vi "ResFileRigExcluder.vi"(7 "Rig Name":string="WT1", 10 "Rig Exclusion Filepath":path=path "/Volumes/CentralDataCache/Projects/GO69T1/Results/KAG69/RigExclusion.xls", 11 "Results file":path=path "/Volumes/CentralDataCache/Projects/GO69T1/Results/KAG69/Profiles2016-08 copy.xls") -> (3 "New Filepath":path=path "/Volumes/CentralDataCache/Projects/GO69T1/Results/KAG69/Profiles2016-08 copy_RigSpec.xls")   [LabVIEW 2016]
doc: "Given {complete Res File, Rig Name, Rig Exclusion Filepath}, this VI returns a Rig-Specific Results File.\n< Rig Name > = relevant Rig Name ; \n< Results File > = comprehensive Results File ; \n< Rig Exclusion Filepath > = path to text file containing list of all Rigs at facility ; \n< New Filepath > = Rig-Specific Results File contains all generic metadata, measurements, and data pertaining to < Rig Name >"
uses:
  Anemometry Sub Vis/Data_plotting_vis/Data_File_Type.ctl
  <vilib>/Utility/file.llb/Read Delimited Spreadsheet (string).vi
  <vilib>/regexp/Match Regular Expression.xnode
panel:
  out "Desired Channels":string[](array[string])=["Date:of:Measurement", "Time:Measurement:Commenced", "Seconds:since:1st Jan", "Measuring:Instrument:Type", "User:Comments:", "Run:Messages:", "Raw:Data:Filename", "Pitot (Uref):X Position:X (mm)", "Pitot (Uref):Y Position:Y (mm)", "Pitot (Uref):Z Position:Z (mm)", "Pitot (Uref):Mean:UREF", "Pitot (Uref):Variance:uref^2", "Pitot (Uref):Standard Error:in Mean", "Pitot (Uref):Timescale Estimate:Integrated to 25%", "Pitot (Uref):Calibration:Filename", "HW (Uhf):X Position:X (mm)", "HW (Uhf):Y Position:Y (mm)", "HW (Uhf):Z Position:Z (mm)", "HW (Uhf):Mean:UHF", "HW (Uhf):Variance:uhf^2", "HW (Uhf):Skewness:uhf^3/(uhf^2)^1.5", "HW (Uhf):Kurtosis:(uhf^4/(uhf^2)^2) -3", "HW (Uhf):Standard Error:in Mean", "HW (Uhf):Standard Error:in Variance", "HW (Uhf):Timescale Estimate:Integrated to 25%", "HW (Uhf):Calibration:Filename", "HW (Uhf):Calibration:Drift", "HW (Uhf):Calibration:Interval", "Av Analogue:Sampling:Rate", "No of:Analogue:Samples", "No Of:Measurement:Blocks", "Flow:Measurement:Time", "Reference:Temperature:Used for Corrections", "Atmos:Pressure:Used for Corrections", "Multi Run:Command:Filename", "Multi Run:Start Time:", "Multi Run:Duration in:Minutes", "Multi Run:Row:Type", "Multi Run:Row:Number", "Multi Run:Extra:Command", "Prog Post:Process:Mode", "Acquisition:PlugIn:Used", "Original:Results:Filename", "Time:According:to", "Client:Seconds:Since", "Averaging:Period:Used", "ADAM:Scan:Time", "Complete:Scan:Period", "Status:of:MetadataSys", "Status:of:Post_Processing_Machine", "CSU:Pressure:mBar", "CSU:Pressure:Age_min", "CFWS:Pressure:mBar", "CFWS:Pressure:Age_min", "CS:AvgPressure:mBar", "WT1:StaticP:0", "WT1:StaticP:1", "WT1:StaticP:2", "WT1:StaticP:3", "WT1:StaticP:4", "WT1:StaticP:5", "WT1:StaticP:6", "WT1:StaticP:7", "WT1:AvStat:P0", "WT1:AvStat:P1", "WT1:AvStat:P2", "WT1:AvStat:P3", "WT1:AvStat:P4", "WT1:AvStat:P5", "WT1:AvStat:P6", "WT1:AvStat:P7", "WT1:Temperature:C", "WT1:Motor:Enable", "WT1:Speed:Calib Tweak", "WT1:Speed:Dem Velocity", "WT1:Speed:Dem Voltage", "WT1:Speed:Meas Velocity", "WT1:Speed:Send Voltage", "WT1:VFD:FREQ", "WT1:RoofSetting:Pressures", "WT1:RoofSetting:Heights", "WT1:Turntable:Azimuth", "WT1Traverse:Motor:X", "WT1Traverse:Motor:Y", "WT1Traverse:Motor:Z", "WT1:Z:Corrections", "WT1 MD:User:Name", "WT1 MD:Project:Number", "WT1 MD:Project:Configuration", "WT1 MD:Pitot:Height", "WT1 MD:Pitot:X-location", "WT1 MD:Roughness:Type", "WT1 MD:Roughness:Size", "WT1 MD:Roughness:AdditionalElements", "WT1 MD:Trip:Height", "WT1 MD:Trip:Location", "WT1 MD:Spires:Type", "WT1 MD:Spires:Code", "WT1 MD:Spires:FullCount", "WT1 MD:Spires:HalfCount", "WT1 MD:Spires:Location", "WT1 MD:Spires:Height", "WT1 MD:Spires:TopWidth", "WT1 MD:Spires:BaseWidth", "WT1 MD:Comments:", "WT1:AQ MD:SourceID", "WT1:Cal Gas:Selector", "WT1:Cal Gas 1:BottleID", "WT1:Cal Gas 1:GasMixture", "WT1:Cal Gas 1:Conc", "WT1:Cal Gas 2:BottleID", "WT1:Cal Gas 2:GasMixture", "WT1:Cal Gas 2:Conc", "WT1:Cal Gas 3:BottleID", "WT1:Cal Gas 3:GasMixture", "WT1:Cal Gas 3:Conc", "WT1:Autozero:Pressures", "ADAM:Scan:Pacer", "WT1:rho:(kg/m^3)", "WT1:FID:IP", "WT1:MFC32:Read%", "WT1:MFC31:Read%", "WT1:MFC25:Read%", "WT1:MFC21:Read%", "WT1:MFC13:Read%", "WT1:MFC12:Read%", "WT1:MFC:Enable", "Status:of:WT1", "WT1 Metadata:Roughness:Notes", "ADAM:Scan:Comments", "Client:ADAM:Scan", "::", "::1904", "::", "::", "::", "::Inc Path", "::", "::", "::", "::", "::", "::Not %", "::(s)", "::", "::", "::", "::", "::", "::", "::", "::", "::Not %", "::Not %", "::(s)", "::", "::%", "::Minutes", "::Freq (Hz)", "::Per Block", "::", "::(mins)", "::", "::", "::", "::", "::", "::", "::", "::", "::", "::", "::", "::Client", "::1st Jan 1904", "::Seconds", "::CPP-ScanTimeKeeper.vi", "::sec", "::", "::", "::", "::CSUWebClient.vi", "::", "::CFWSWebClient.vi", "::", "::CSPressureSelector.vi", "::", "::", "::", "::", "::", "::", "::", "::", ":: WT1", ":: WT1", ":: WT1", ":: WT1", ":: WT1", ":: WT1", ":: WT1", ":: WT1", "::", "::LabJackT7.vi", "::", "::", "::WT1", "::WT1", "::", "::", "::", "::", "::", "::", "::", "::", "::", "::", "::", "::None", "::1000.0 mm", "::-3350.0 mm", "::0.0-mm None + None", "::0.0-mm None", "::98", "::0.0 mmModified 09-08-2016 21", "::0.0 mm", "::Irwin", "::24X4", "::0 full", "::0 half", "::0.0 mm", "::609.6 mm", "::0.0 mm", "::101.6 mm", "::NEW 1.5in roughness", "::", "::", "::", "::", "::", "::", "::", "::", "::", "::", "::", "::", "::", "::", "::", "::", "::", "::", "::", "::", "::", "::", "::", "::", "::", "::", "::", "::", "::", "::", "::", "::", "::", "::UINT16", "::UINT16", "::UINT16", "::UINT16", "::UINT16", "::UINT16", "::UINT16", "::UINT16", "::", "::", "::", "::", "::", "::", "::", "::", "::", "::", "::", "::", "::", "::", "::", "::", "::", "::", "::", "::A", "::1000.0 mm", "::-3532.0 mm", "::50.8-mm Cubes + 98", "::50.8-mm Cubes", "::98", "::558.8 mm", "::527.0 mm", "::Irwin", "::72X5", "::4 full", "::2 half", "::223.8 mm", "::1828.8 mm", "::44.4 mm", "::133.3 mm", "::(add comments)", "::", "::", "::100.00 inches", "::200.00 inches", "::100.00 inches", "::-50.00 inches", "::0.00 inches", "::RE-run of 413... this time with gases on!! (10x20x10cm EBD w/ stack in center)", "::", "::", "::", "::", "::", "::", "::", "::", "::", "::", "::", "::", "::", "::", "::", "::", "::", "::", "::", "::", "::", "::", "::", "::", "::", "::", "::A", "::1000.0 mm", "::-3532.0 mm", "::50.8-mm Cubes + 98", "::50.8-mm Cubes", "::98", "::558.8 mm", "::527.0 mm", "::Irwin", "::72X5", "::4 full", "::2 half", "::223.8 mm", "::1828.8 mm", "::44.4 mm", "::133.3 mm", "::(add comments)", "::", "::", "::", "::", "::", "::", "::", "::", "::", "::", "::", "::", "::", "::", "::", "::", "::", "::", "::", "::", "::", "::", "::", "::", "::", "::", "::", "::", "::", "::", "::", "::", "::", "::", "::", "::", "::", "::", "::", "::", "::", "::", "::Xdim", "::Ydim (mm)", "::Zdim (mm)", "::(mm)", "::(mm)", "::", "::(add comments)", "::", "::", "::", "::", "::", "::", "::", "::", "::", "::", "::", "::", "::", "::", "::", "::", "::", "::", "::", "::", "::", "::", "::", "::", "::", "::", "::", "::", "::Fr Server", "::Comments"]
  out "Desired Columns":i32[](array[numeric])=[0, 1, 2, 3, 4, 5, 6, 7, 8, 9, 10, 11, 12, 13, 14, 15, 16, 17, 18, 19, 20, 21, 22, 23, 24, 25, 26, 27, 28, 29, 30, 31, 32, 33, 34, 35, 36, 37, 38, 39, 40, 41, 42, 43, 44, 45, 46, 47, 48, 49, 51, 52, 53, 54, 55, 56, 57, 58, 59, 60, 61, 62, 63, 64, 65, 66, 67, 68, 69, 70, 71, 72, 73, 74, 75, 76, 77, 78, 79, 80, 81, 82, 83, 84, 85, 86, 87, 88, 89, 90, 91, 92, 93, 94, 95, 96, 97, 98, 99, 100, 101, 102, 103, 104, 105, 106, 107, 108, 109, 110, 111, 112, 113, 114, 115, 116, 261, 266, 285, 287, 298, 299, 300, 301, 302, 303, 304, 322, 323, 324, 325, 326, 327, 328, 329, 330, 331, 332, 333, 334, 335, 336, 337, 338, 339, 340, 341, 342, 343, 344, 345, 346, 347, 348, 349, 350, 351, 352, 353, 354, 355, 356, 357, 358, 359, 360, 361, 362, 363, 364, 365, 366, 367, 368, 369, 370, 371, 372, 373, 374, 375, 376, 377, 378, 379, 380, 381, 382, 383, 384, 385, 386, 387, 388, 389, 390, 391, 392, 393, 394, 395, 396, 397, 398, 399, 400, 401, 402, 403, 404, 405, 406, 407, 408, 409, 410, 411, 412, 413, 414, 415, 416, 417, 418, 419, 420, 421, 422, 423, 424, 425, 426, 427, 428, 429, 430, 431, 432, 433, 434, 435, 436, 437, 438, 439, 440, 441, 442, 443, 444, 445, 446, 447, 448, 449, 450, 451, 462, 463, 464, 465, 468, 469, 470, 471, 472, 473, 474, 475, 476, 477, 478, 479, 480, 481, 482, 483, 484, 485, 486, 487, 488, 489, 490, 491, 492, 493, 494, 495, 496, 497, 498, 499, 500, 501, 502, 503, 504, 505, 506, 507, 508, 509, 510, 511, 512, 513, 514, 515, 516, 517, 518, 519, 520, 521, 522, 523, 524, 525, 526, 527, 528, 529, 530, 531, 532, 533, 534, 535, 536, 537, 538, 539, 540, 541, 542, 543, 544, 545, 546, 547, 548, 549, 550, 551, 552, 553, 554, 555, 556, 557, 558, 559, 560, 561, 562, 563, 564, 565, 566, 567, 568, 569, 570, 571, 572, 573, 574, 575, 576, 577, 578, 579, 580, 581, 582, 583, 584, 585, 586, 587, 588, 589, 591, 592, 593, 594, 595, 596, 597, 598, 599, 600, 601, 602, 603, 604, 605, 606, 607, 608, 609, 610, 611, 612, 613, 614, 615, 616, 617, 618, 619, 620, 621, 622, 623, 624, 625, 626, 627, 628, 629, 630, 631, 632, 633, 634, 635, 636, 637, 638, 639, 640, 641, 642, 643, 644, 645, 646, 647, 648, 649, 650]
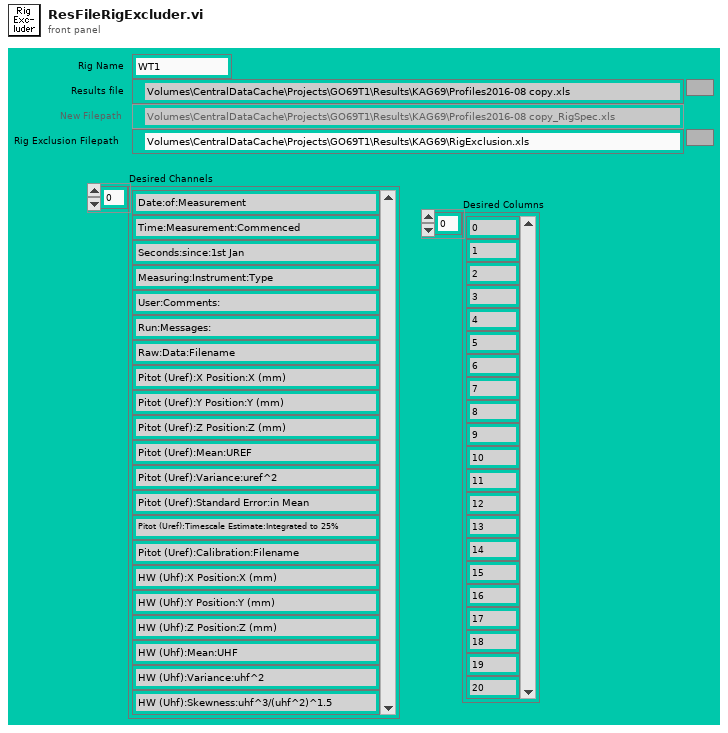
[diagram p1: front panel]
types:
  T1 = enum16{"Show only data summary", "Show data summary", "No data summary"}
  T2 = typedef "Data_File_Type.ctl" = enum16{"Read All File Types", "Results Files Only", "Raw Data Files Only", "Calibration Files Only", "Gas Desk Files Only", "Old Results Files Only", "Tabulated Data Files Only"}
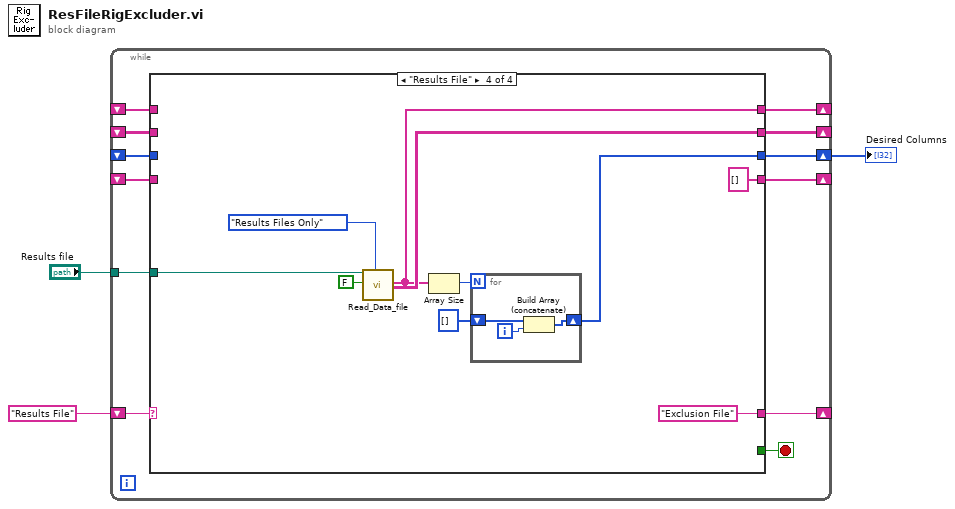
[diagram p0: block diagram]
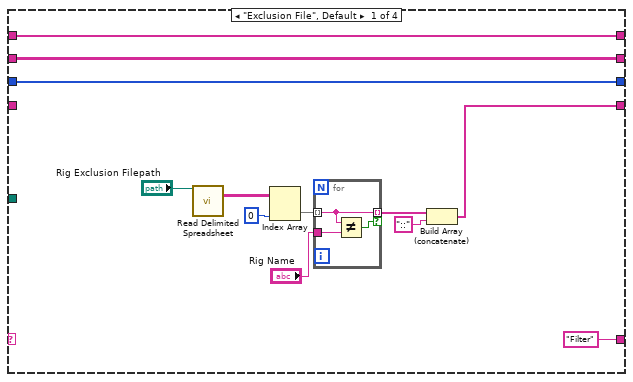
[diagram p2: hidden frame]
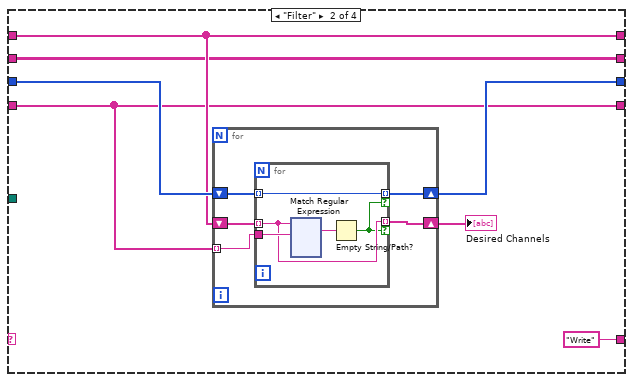
[diagram p3: hidden frame]
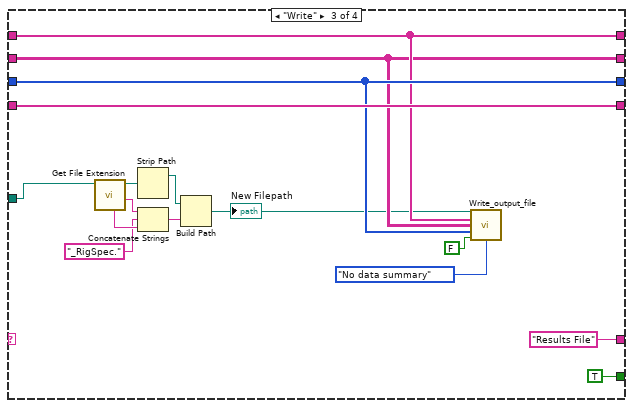
[diagram p4: hidden frame]
diagram:
  n1 = while {
    shift-right: [w14] -> _
    shift-left: "Results File" -> [w15]
    shift-right: [w12] -> _
    shift-left: _ -> [w11]
    shift-right: [w10] -> _
    shift-left: _ -> [w9]
    shift-right: [w8] -> w1
    shift-left: _ -> [w7]
    shift-right: [w6] -> _
    shift-left: _ -> [w5]
    tunnel: "Results file" -> [w4]
    stop <- w13 stop-if-true
    n2 = case shown="\"Results File\"" w15 {
      tunnel: ["Filter" "Write" "Results File" "Exclusion File"] -> w14
      tunnel: [_ _ TRUE _] -> w13
      tunnel: [w17 w33 w164 w183] -> w12
      tunnel: w11 -> [w17 w33 w164 _]
      tunnel: [w18 w34 w165 w182] -> w10
      tunnel: w9 -> [w18 w34 w165 _]
      tunnel: [w16 w35 w167 w181] -> w8
      tunnel: w7 -> [w16 w36 w167 _]
      tunnel: [w19 w32 w168 string[] []] -> w6
      tunnel: w5 -> [_ w32 w168 _]
      tunnel: w4 -> [_ _ w170 w179]
      frame "Exclusion File", Default {
        n3 = call-poly <vilib>:"Read Delimited Spreadsheet.vi"("file path (dialog if empty)"="Rig Exclusion Filepath") -> ("all rows"=w21:string[][])  [unwired: 9 in, 5 out]
        n4 = Index Array(array=w21, index (col)=0 ("disabled index (col)")) -> (element=w23:string[])  [unwired: 1 in]
        n5 = for {
          tunnel: w23 -> [w29] mode=indexing
          tunnel: "Rig Name" -> [w30]
          tunnel: [w29] -> w25 mode=indexing if=w28
          n6 = Not Equal?(x=w29, y=w30) -> (x != y?=w28:bool)
        }
        n7 = Build Array (concatenate)(w25, "::" ("array")) -> (w19:string[])
      }
      frame "Filter" {
        n8 = for {
          tunnel: w32 -> [w41] mode=indexing
          shift-right: [w40] -> w31
          shift-left: w34 -> [w42]
          shift-right: [w39] -> w35
          shift-left: w36 -> [w38]
          n9 = for {
            tunnel: w41 -> [w47]
            tunnel: w42 -> [w45] mode=indexing
            tunnel: [w43] -> w39 mode=indexing if=w44
            tunnel: [w45] -> w40 mode=indexing if=w44
            tunnel: w38 -> [w43] mode=indexing
            n10 = xnode "Match Regular Expression"("input string"=w45, "regular expression"=w47) -> ("whole match"=w46:string)  [unwired: 4 in, 4 out]
            n11 = Empty String/Path?(string/path=w46) -> (empty?=w44:bool)
          }
        }
        "Desired Channels" <- w31
      }
      frame "Write" {
        n12 = call <vilib>:"Get File Extension.vi"("file"=w170) -> ("filename without extension"=w171:string, "dup file"=w163:path, "unmodified file extension"=w173:string)  [unwired: 6 in, 2 out]
        n13 = Strip Path(path=w163) -> (stripped path=w174:path)  [unwired: 1 out]
        n14 = Concatenate Strings(w171, "_RigSpec." ("string"), w173) -> (w175:string)
        n15 = Build Path(base path=w174, name or relative path=w175) -> (appended path=w162:path)
        "New Filepath" <- w162
        n16 = call "Write_output_file.vi"("Output filename"=w162, "Channel Names"=w165, "Data"=w164, "Desired Columns"=w167, "Simple Save?"=FALSE, "Summarise mode"=T1."No data summary") -> ()  [unwired: 6 in, 4 out]
      }
      frame "Results File" {
        n17 = call "Read_Data_file.vi"("Results file"=w179, "Delete First Rows?"=FALSE, "Desired File Types"=Data_File_Type."Results Files Only") -> ("Ch names Out"=w182:string[], "Channel Values Out"=w183:string[][])  [unwired: 3 in, 12 out]
        n18 = Array Size(array=w182) -> (size(s)=w184:i32)
        n19 = for {
          N: w184 -> [_]
          shift-right: [w190] -> w181
          shift-left: i32[] [] -> [w189]
          i -> [w188]
          n20 = Build Array (concatenate)(w189, w188) -> (w190:i32[])
        }
      }
    }
  }
  "Desired Columns" <- w1
